vi "Get Updated Path If Necessary.vi"(9 "New Name":string, 11 "Original Path":path) -> (1 "Update?":bool, 3 "New Path":path)   [LabVIEW 2020, in "ADAS_IO_Template_MDO.lvclass"]
uses:
  ADAS_IO_Template_MDO.lvclass
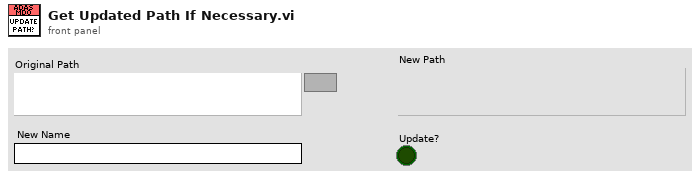
[diagram p1: front panel]
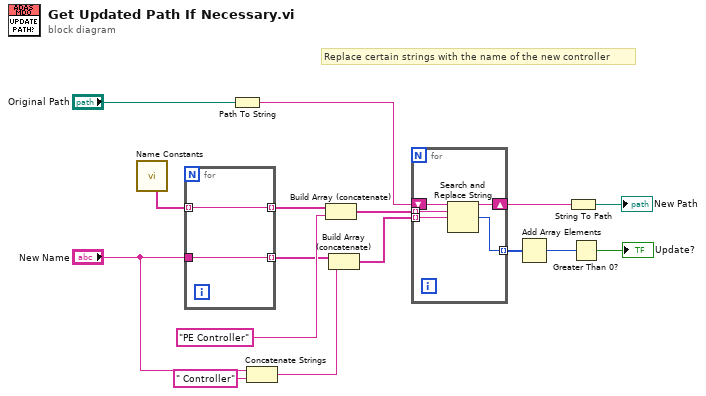
[diagram p0: block diagram]
diagram:
  # "Replace certain strings with the name of the new controller"
  n1 = call "Name Constants.vi"() -> ("Strings to Replace w Name"=w9:string[])  [unwired: 9 in, 2 out]
  n2 = for {
    tunnel: w9 -> [w18] mode=indexing
    tunnel: "New Name" -> [w17]
    tunnel: [w18] -> w6 mode=indexing
    tunnel: [w17] -> w3 mode=indexing
  }
  n3 = Path To String(path="Original Path") -> (string=w15:string)
  n4 = Concatenate Strings("New Name", " Controller" ("string")) -> (w1:string)
  n5 = Build Array (concatenate)(w6, "PE Controller") -> (w5:string[])
  n6 = Build Array (concatenate)(w3, w1) -> (w2:string[])
  n7 = for {
    tunnel: w5 -> [w22] mode=indexing
    tunnel: [w21] -> w12 mode=indexing
    tunnel: w2 -> [w19] mode=indexing
    shift-right: [w20] -> w14
    shift-left: w15 -> [w23]
    n8 = Search and Replace String(input string=w23, search string=w22, replace string=w19) -> (result string=w20:string, number of replacements=w21:i32)  [unwired: 5 in, 2 out]
  }
  n9 = Add Array Elements(numeric array=w12) -> (sum=w11:i32)
  n10 = String To Path(string=w14) -> (path=→"New Path":path)
  n11 = Greater Than 0?(x=w11) -> (x > 0?=→"Update?":bool)
